vi "Initialize Instrument Attribute.vi"(7 "Attribute.Instrument in":refnum<class "Attribute.Instrument.lvclass">) -> (3 "Attribute.Instrument out":refnum<class "Attribute.Instrument.lvclass">)   [LabVIEW 2019, in "Instrument Attributes.lvlib" / "Attribute.Instrument.lvclass"]
uses:
  Attribute.Instrument.lvclass
  C:/Program Files (x86)/National Instruments/LabVIEW 2019/vi.lib/JKI/JKI SMO/Support/Attribute/Attribute.lvclass
  <vilib>/JKI/JKI SMO/Definitions/def.SMO/Scope -- Enum.ctl
  <vilib>/JKI/JKI SMO/Support/Attribute/Attribute.lvclass/Attribute.ctl
  Attribute.Instrument.lvclass/Attribute.Instrument.ctl
  <vilib>/JKI/JKI SMO/Support/Attribute/Attribute.lvclass
  <vilib>/JKI/JKI SMO/Definitions/def.SMO/def.SMO.lvclass
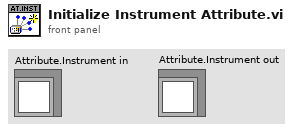
[diagram p1: front panel]
types:
  T1 = typedef "def.SMO.lvclass/Scope -- Enum.ctl" = enum16{"Public", "Protected", "Private"}
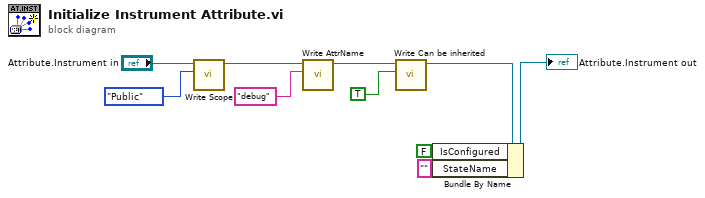
[diagram p0: block diagram]
diagram:
  n1 = call <vilib>:"Write Scope.vi"("Scope"=Scope_--_Enum."Public", "Attribute in"="Attribute.Instrument in") -> ("Attribute out"=w8:refnum<class "Attribute.Instrument.lvclass">)  [unwired: 9 in]
  n2 = call <vilib>:"Write AttrName.vi"("Attribute Name"="debug", "Attribute in"=w8) -> ("Attribute out"=w5:refnum<class "Attribute.Instrument.lvclass">)  [unwired: 9 in]
  n3 = call <vilib>:"Write Can be inherited.vi"("Can be inherited"=TRUE, "Attribute in"=w5) -> ("Attribute out"=w4:refnum<class "Attribute.Instrument.lvclass">)  [unwired: 8 in, 1 out]
  n4 = Bundle By Name(cluster=w4, "IsConfigured"=FALSE ("isInstalled"), "StateName"="" ("state")) -> (→"Attribute.Instrument out":refnum<class "Attribute.Instrument.lvclass">)
